vi "外观 1.vi"(0 "Data In":T1 {"仪器时间" format="%<%Y/%m/%d %H:%M:%S>T"; "门状态" items=["关闭", "打开"]; "采样模式" items=["定时留样"=1, "时间等比"=2, "同步留样"=3, "外控留样"=4, "超标留样"=5]; "工作进程" items=["停止中"=0, "启动延时"=1, "外置泵延时"=2, "管路润洗"=3, "管存"=4, "留样"=5, "出水管路排空"=6, "采水管路排空"=7, "待机"=13]; "工作状态" items=["停止", "运行", "系统初始化"]}, 2 "Display State In":T4 caption="显示状态输入", 3 "Container State":T5 caption="容器状态") -> (6 "Data Out":T2 {"仪器时间" format="%<%Y/%m/%d %H:%M:%S>T"; "门状态" items=["关闭", "打开"]; "采样模式" items=["定时留样"=1, "时间等比"=2, "同步留样"=3, "外控留样"=4, "超标留样"=5]; "工作进程" items=["停止中"=0, "启动延时"=1, "外置泵延时"=2, "管路润洗"=3, "管存"=4, "留样"=5, "出水管路排空"=6, "采水管路排空"=7, "待机"=13]; "工作状态" items=["停止", "运行", "系统初始化"]}, 7 "Display State Out":T4 caption="显示状态输出", 8 "Action":T3 caption="动作")   [LabVIEW 2016, in "德润超标留样.lvlib" / "超标留样运行状态.xctl"]
uses:
  <vilib>/_xctls/Container State.ctl
  <vilib>/_xctls/Action.ctl
  <vilib>/_xctls/XControlSupport.lvlib
panel:
  out "当前瓶号":string
  out "采样瓶数":string
  out "采样模式":string
  out "测量模式":string
  out "工作状态":string
  out "仪器时间":string
  # "当前瓶号:"
  # "仪器时间:"
  # "工作状态:"
  # "测量模式:"
  # "采样模式:"
  # "采样瓶数:"
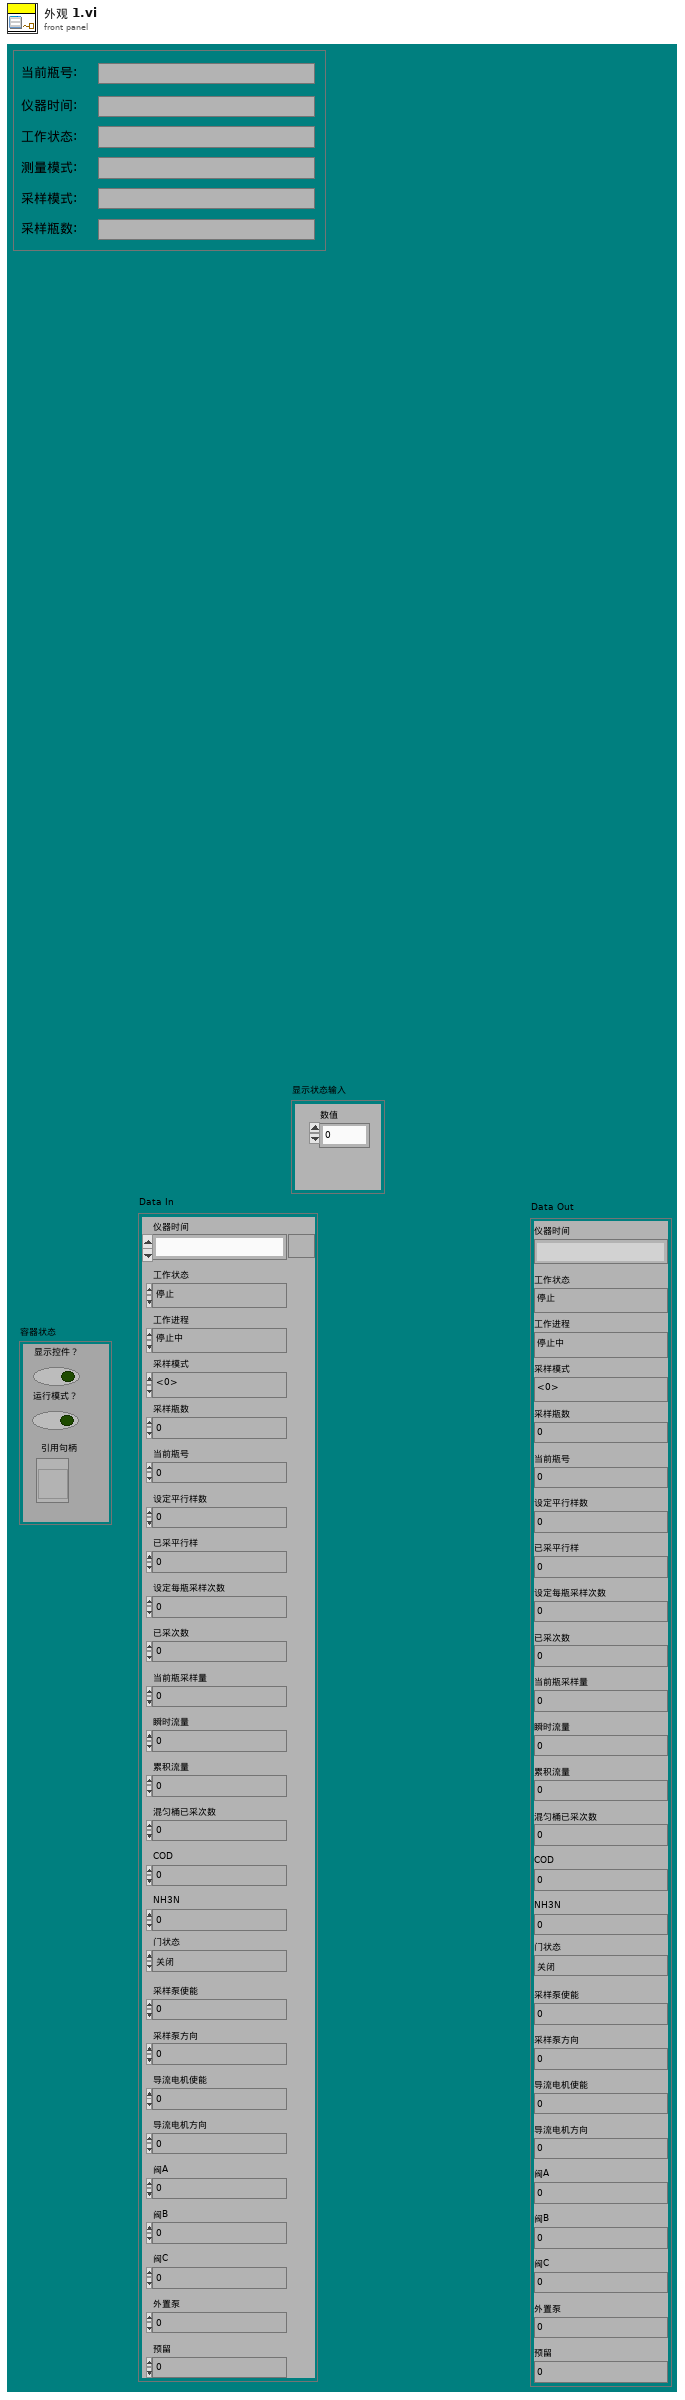
[diagram p1: front panel]
types:
  T1 = typedef "德润超标留样.lvlib/超标留样运行状态.xctl/数据 1.ctl" = cluster{"仪器时间":timestamp, "工作状态":u16, "工作进程":u16, "采样模式":u16, "采样瓶数":dbl, "当前瓶号":dbl, "设定平行样数":dbl, "已采平行样":dbl, "设定每瓶采样次数":dbl, "已采次数":dbl, "当前瓶采样量":dbl, "瞬时流量":dbl, "累积流量":dbl, "混匀桶已采次数":dbl, "COD":dbl, "NH3N":dbl, "门状态":u16, "采样泵使能":dbl, "采样泵方向":dbl, "导流电机使能":dbl, "导流电机方向":dbl, "阀A":dbl, "阀B":dbl, "阀C":dbl, "外置泵":dbl, "预留":dbl}
  T2 = cluster{"仪器时间":timestamp, "工作状态":u16, "工作进程":u16, "采样模式":u16, "采样瓶数":dbl, "当前瓶号":dbl, "设定平行样数":dbl, "已采平行样":dbl, "设定每瓶采样次数":dbl, "已采次数":dbl, "当前瓶采样量":dbl, "瞬时流量":dbl, "累积流量":dbl, "混匀桶已采次数":dbl, "COD":dbl, "NH3N":dbl, "门状态":u16, "采样泵使能":dbl, "采样泵方向":dbl, "导流电机使能":dbl, "导流电机方向":dbl, "阀A":dbl, "阀B":dbl, "阀C":dbl, "外置泵":dbl, "预留":dbl}
  T3 = typedef "XControlSupport.lvlib/Action.ctl" = cluster{"Data Changed?":bool, "State Changed?":bool, "Action Name":string}
  T4 = typedef "德润超标留样.lvlib/超标留样运行状态.xctl/状态 2.ctl" = cluster{"Numeric":dbl}
  T5 = typedef "XControlSupport.lvlib/Container State.ctl" = cluster{"Indicator?":bool, "Run Mode?":bool, " Refnum":refnum<vi>}
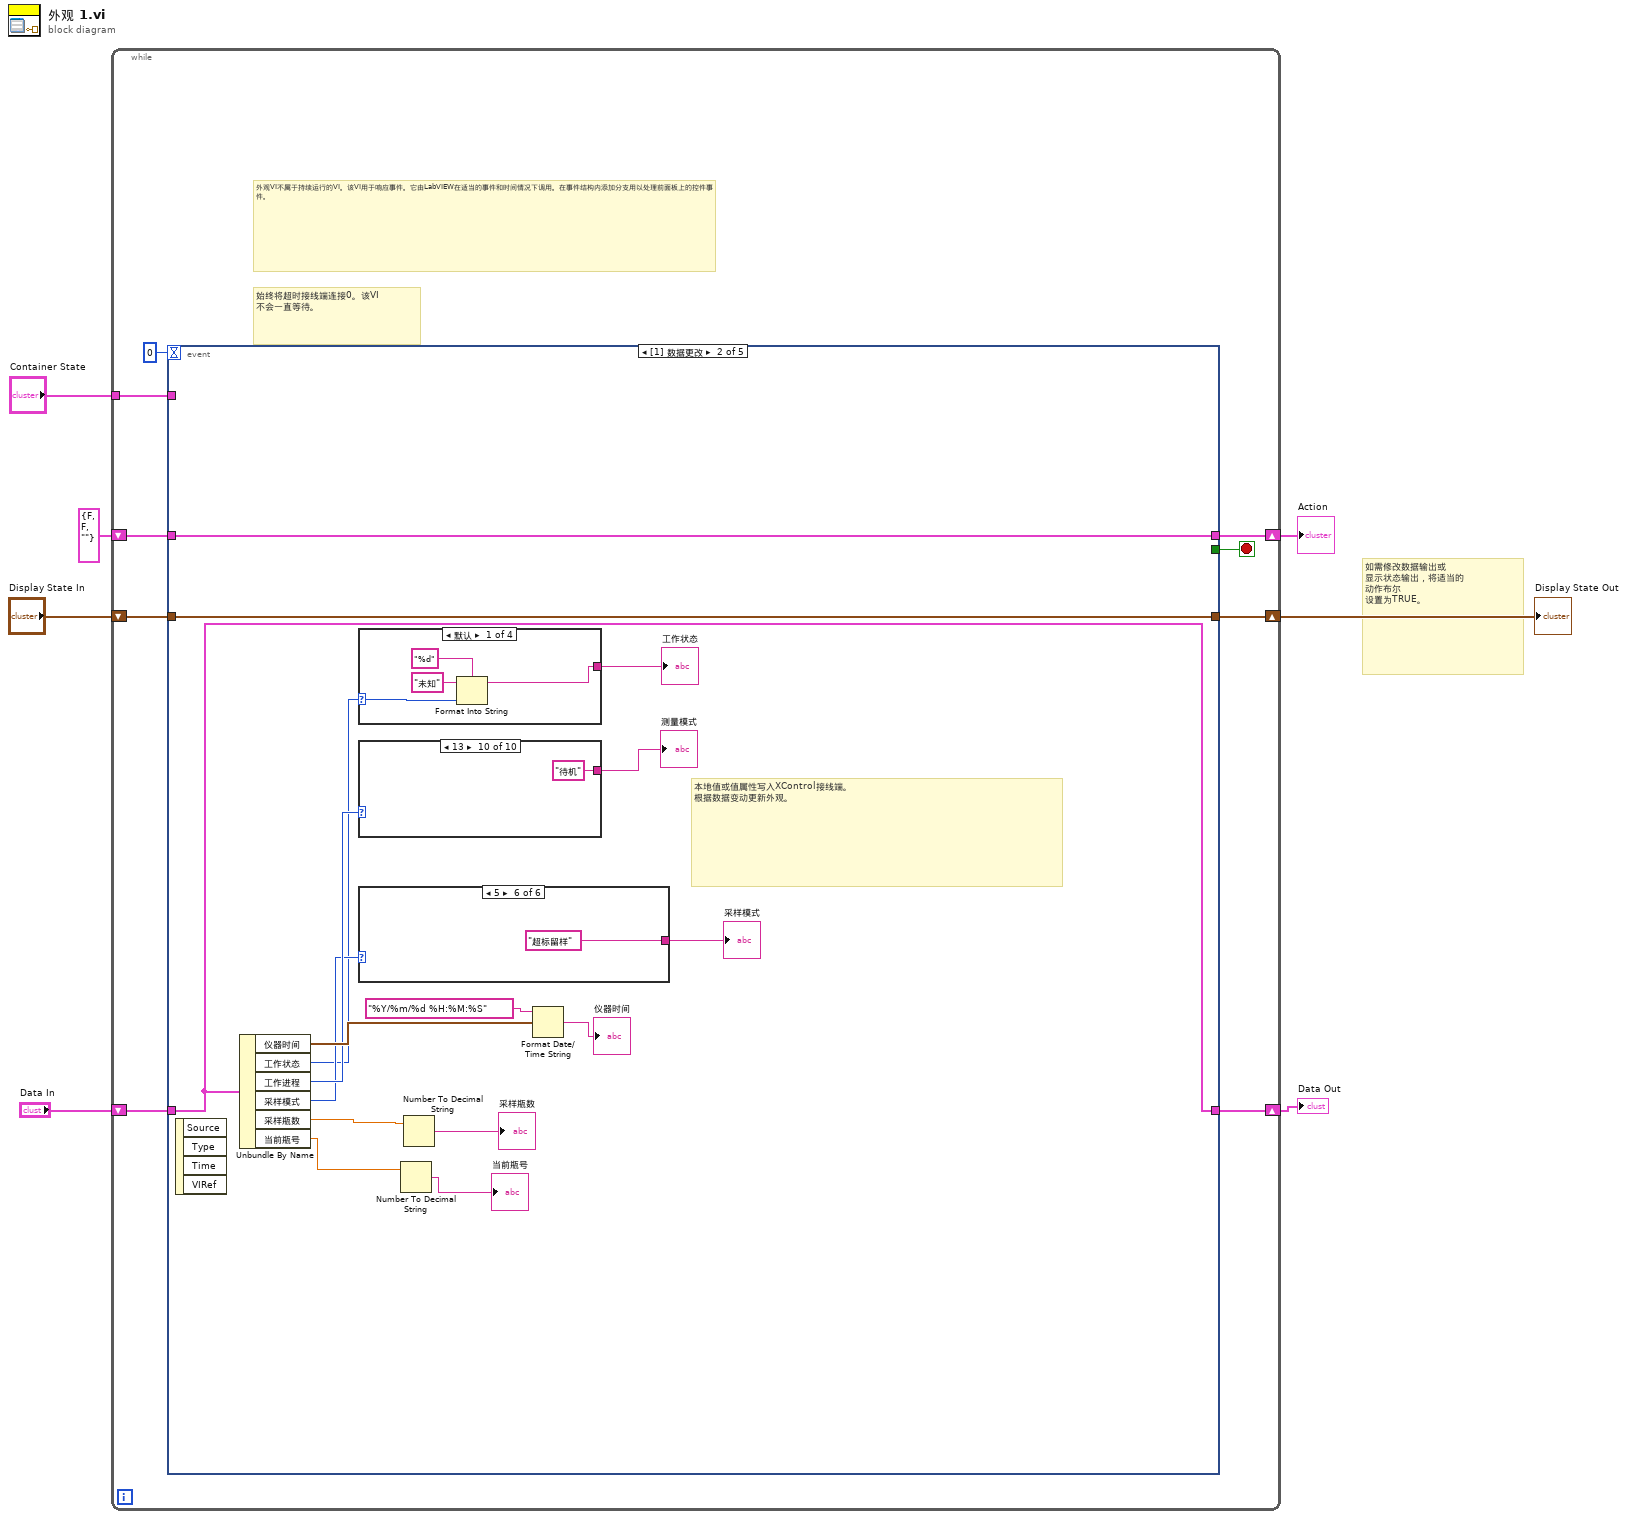
[diagram p0: block diagram]
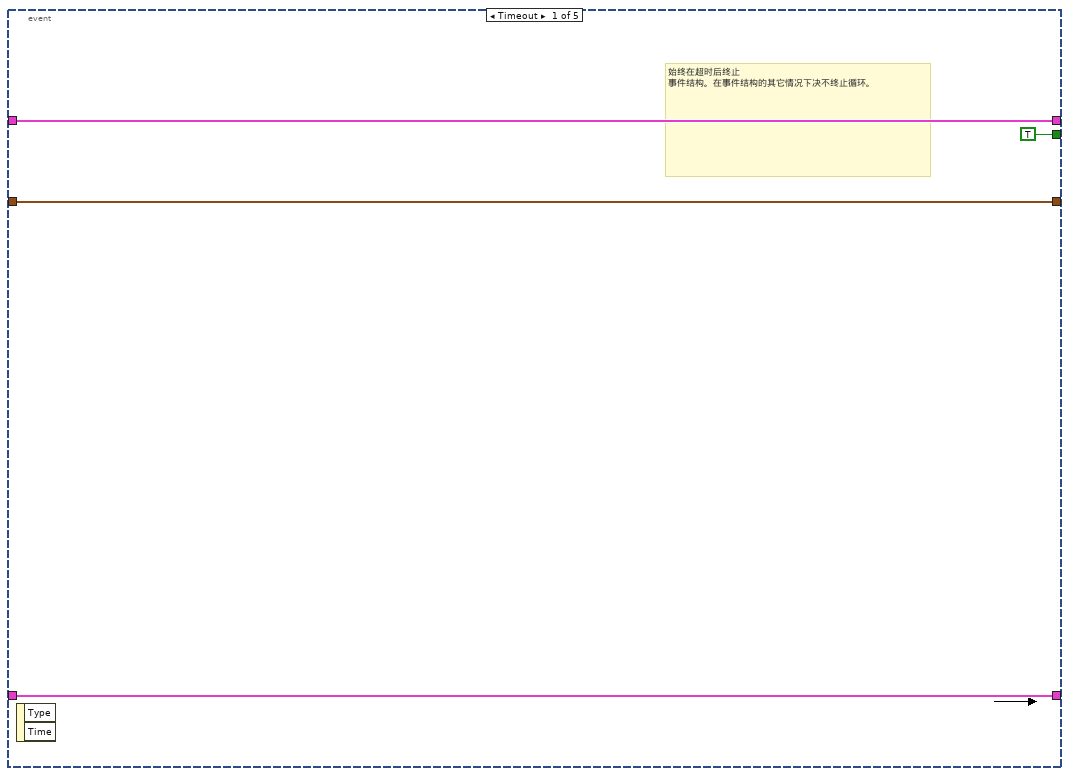
[diagram p2: hidden frame]
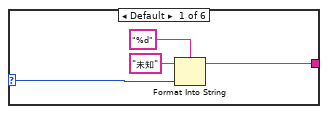
[diagram p3: hidden frame]
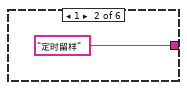
[diagram p4: hidden frame]
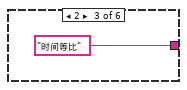
[diagram p5: hidden frame]
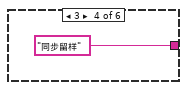
[diagram p6: hidden frame]
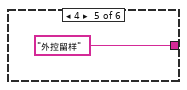
[diagram p7: hidden frame]
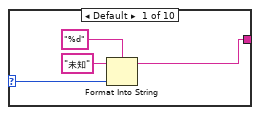
[diagram p8: hidden frame]
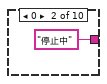
[diagram p9: hidden frame]
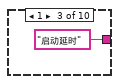
[diagram p10: hidden frame]
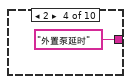
[diagram p11: hidden frame]
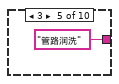
[diagram p12: hidden frame]
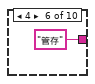
[diagram p13: hidden frame]
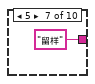
[diagram p14: hidden frame]
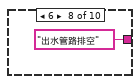
[diagram p15: hidden frame]
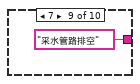
[diagram p16: hidden frame]
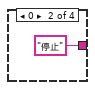
[diagram p17: hidden frame]
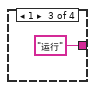
[diagram p18: hidden frame]
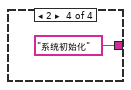
[diagram p19: hidden frame]
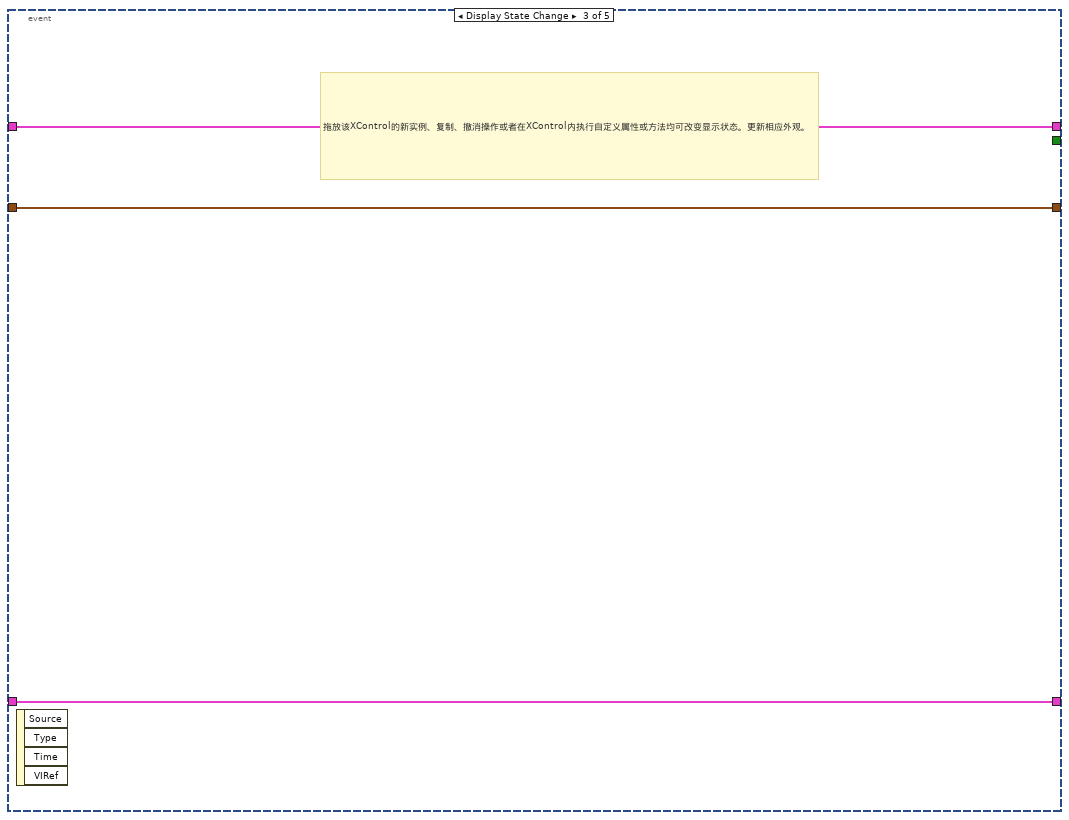
[diagram p20: hidden frame]
diagram:
  # "如需修改数据输出或\n显示状态输出，将适当的\n动作布尔\n设置为TRUE。"
  n1 = while {
    shift-right: [w15] -> w6
    shift-left: "Display State In" -> [w16]
    tunnel: "Container State" -> [w12]
    shift-right: [w10] -> w2
    shift-left: "Data In" -> [w11]
    shift-right: [w8] -> w4
    shift-left: T3 {"Data Changed?"=FALSE, "State Changed?"=FALSE, "Action Name"=""} ("Action") -> [w9]
    stop <- w14 stop-if-true
    # "外观VI不属于持续运行的VI。该VI用于响应事件。它由LabVIEW在适当的事件和时间情况下调用。在事件结构内添加分支用以处理前面板上的控件事件。"
    # "始终将超时接线端连接0。该VI\n不会一直等待。"
    n2 = event shown="[1] 数据更改" {
      selector: _ -> [_ _ _ _ _]
      dyn-events: _ -> [_ _ _ _ _]
      timeout: 0 -> [_ _ _ _ _]
      tunnel: w16 -> [w18 w36 w68 w71 w75]
      tunnel: [w18 w36 w68 w71 w75] -> w15
      tunnel: [TRUE _ _ _ _] -> w14
      tunnel: w12 -> [_ _ _ w72 w76]
      tunnel: w11 -> [w17 w34 w67 w70 w74]
      tunnel: [w17 w34 w67 w70 w74] -> w10
      tunnel: [w19 w35 w66 w69 w73] -> w8
      tunnel: w9 -> [w19 w35 w66 w69 w73]
      event Timeout {
        # "始终在超时后终止\n事件结构。在事件结构的其它情况下决不终止循环。"
        n3 = event-data() -> ()  [unwired: 1 in, 2 out]
      }
      event Data Change {
        # "本地值或值属性写入XControl接线端。\n根据数据变动更新外观。"
        n4 = event-data() -> ()  [unwired: 1 in, 4 out]
        n5 = Unbundle By Name(w34) -> ("仪器时间"=w32:timestamp, "工作状态"=w25:u16, "工作进程"=w29:u16, "采样模式"=w27:u16, "采样瓶数"=w24:dbl, "当前瓶号"=w22:dbl)
        n6 = case shown="默认" w25 {
          selector: w25 -> [w59 _ _ _]
          tunnel: [w60 "停止" ("工作状态") "运行" ("工作状态") "系统初始化" ("工作状态")] -> w30
          frame Default {
            n7 = Format Into String(format string="%d" ("格式字符串"), initial string="未知" ("工作状态"), w59) -> (resulting string=w60:string)  [unwired: 1 in, 1 out]
          }
          frame 0 {
          }
          frame 1 {
          }
          frame 2 {
          }
        }
        "工作状态" <- w30
        n8 = case shown="13" w29 {
          selector: w29 -> [w46 _ _ _ _ _ _ _ _ _]
          tunnel: [w47 "停止中" "启动延时" "外置泵延时" "管路润洗" "管存" "留样" "出水管路排空" "采水管路排空" "待机"] -> w28
          frame Default {
            n9 = Format Into String(format string="%d" ("格式字符串"), initial string="未知" ("工作状态"), w46) -> (resulting string=w47:string)  [unwired: 1 in, 1 out]
          }
          frame 0 {
          }
          frame 1 {
          }
          frame 2 {
          }
          frame 3 {
          }
          frame 4 {
          }
          frame 5 {
          }
          frame 6 {
          }
          frame 7 {
          }
          frame 13 {
          }
        }
        "测量模式" <- w28
        n10 = case shown="5" w27 {
          selector: w27 -> [w38 _ _ _ _ _]
          tunnel: [w37 "定时留样" "时间等比" "同步留样" "外控留样" "超标留样"] -> w26
          frame Default {
            n11 = Format Into String(format string="%d" ("格式字符串"), initial string="未知" ("工作状态"), w38) -> (resulting string=w37:string)  [unwired: 1 in, 1 out]
          }
          frame 1 {
          }
          frame 2 {
          }
          frame 3 {
          }
          frame 4 {
          }
          frame 5 {
          }
        }
        "采样模式" <- w26
        n12 = Number To Decimal String(number=w22) -> (decimal integer string=→"当前瓶号":string)  [unwired: 1 in]
        n13 = Number To Decimal String(number=w24) -> (decimal integer string=→"采样瓶数":string)  [unwired: 1 in]
        n14 = Format Date/Time String(time format string (%c)="%Y/%m/%d %H:%M:%S" ("时间格式字符串(%c)"), seconds (now)=w32) -> (date/time string=→"仪器时间":string)  [unwired: 1 in]
      }
      event Display State Change {
        # "拖放该XControl的新实例、复制、撤消操作或者在XControl内执行自定义属性或方法均可改变显示状态。更新相应外观。"
        n15 = event-data() -> ()  [unwired: 1 in, 4 out]
      }
      event Direction Change {
        # "XControl的方向由输入控件转换为显示控件，反之亦然。更新相应外观。"
        n16 = event-data() -> ()  [unwired: 1 in, 4 out]
        n17 = Unbundle By Name(w72) -> ()  [unwired: 1 out]
      }
      event Exec State Change {
        # "包含该XControl的VI已从编辑模式切换至运行模式，反之亦然。\n相应的更新外观。"
        # "分别处理编辑模式和\n运行模式"
        n18 = event-data() -> ()  [unwired: 1 in, 4 out]
        n19 = Unbundle By Name(w76) -> ()  [unwired: 1 out]
      }
    }
  }
  "Display State Out" <- w6
  "Action" <- w4
  "Data Out" <- w2
